vi "Change AO Gain On Fly or Not On Fly.vi"() -> ()   [LabVIEW 2015]
doc: "I. Description:\nThis example demonstrates how to output a continuous periodic waveform using an internal sample clock.\n\nII. Instructions for Running:\n1. Select the Physical Channel to correspond to where your signal is output on the DAQ device.\n2. Enter the Minimum and Maximum Voltage Ranges\n3. Specify the Desired Frequency of the output Waveform\n4. Enter the Waveform Information. See the documentation of the Waveform Buffer Generation SubVI for information on each parameter.\n\nIII. Block Diagram Steps:\n1. Create an Analog Output Voltage channel.\n2. Call the DAQmx Timing (Use Waveform) VI which sets the sample clock rate based on the input waveform parameters, and set the sample mode to Continuous.\n3. Write the waveform to the output buffer.\n4. Call the Start VI.\n5. Loop continuously until the user presses the Stop button. Check for errors every 100 ms using the Is Task Done? VI\n6. Clear the Task\n7. Use the popup dialog box to display an error or warning if any.\n\nIV. I/O Connections Overview:\nMake sure your signal output terminal matches the Physical Channel I/O Control. For further connection information, refer to your hardware reference manual."
uses:
  <vilib>/DAQmx/create/channels.llb/DAQmx Create Channel (AO-Voltage-Basic).vi
  <vilib>/Utility/error.llb/DialogType.ctl
  <vilib>/DAQmx/configure/timing.llb/DAQmx Timing (Sample Clock).vi
  <vilib>/DAQmx/write.llb/DAQmx Write (Analog 2D DBL NChan NSamp).vi
  <resource>/objmgr/daqmx.rc
panel:
  in  "Gain property node":i32
  in  "physical channels 2":tag="PXI1Slot2/ao0" caption="Output Physical Channels"
  in  "AO Idle State":bool=TRUE
  in  "Gain Setting 2":u16(ring) items=["0 dB Gain"=0, "20 dB Gain"=2, "40 dB Gain"=4]
  in  "AO Channel 2":u16(ring)=1536 items=["AO 0"=1536, "AO 1"=1540]
  in  "AO Channel":u16(ring)=1536 items=["AO 0"=1536, "AO 1"=1540]
  in  "Gain Setting":u16(ring) items=["0 dB Gain"=0, "20 dB Gain"=2, "40 dB Gain"=4]
  out "Resulting Frequency":dbl format="%.2f"
  in  "Cycles per Buffer":i32=5
  in  "Waveform Type":T1(ring)
  in  "Desired Frequency":dbl=1000.0 format="%.2f"
  in  "Samples per Buffer":dbl=250.0
  in  "Amplitude":dbl=1750000000.0 format="%0.2p"
  out "Waveform Graph":dbl[](graph) caption="Output Waveform"
  in  "Physical Channels":tag="PXI1Slot2/ao0:1"
  in  "Minimum Value":dbl=-10.0 format="%0.2f"
  in  "Maximum Value":dbl=10.0 format="%0.2f"
  in  "stop":bool
  # "For instructions, select Help>>Show Context Help"
  # "Channel Parameters"
  # "Timing Parameters"
  # "Waveform Information"
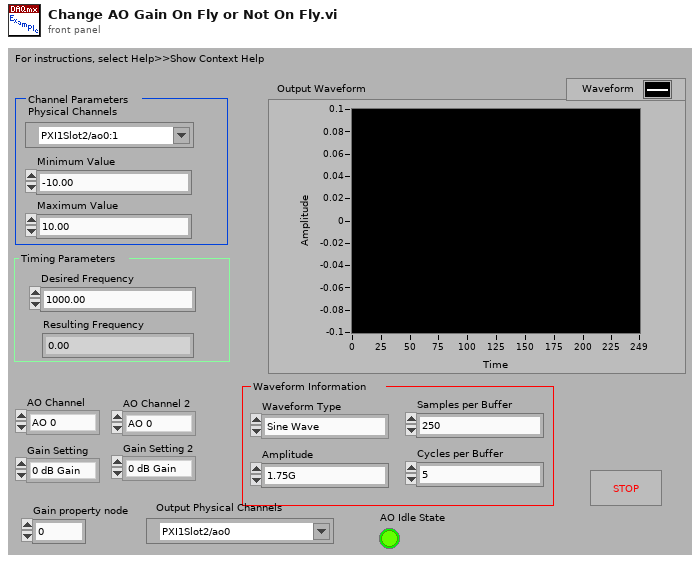
[diagram p1: front panel]
types:
  T1 = enum16{"Sine Wave", "Triangle Wave", "Square Wave", "Sawtooth Wave"}
  T2 = typedef "DialogType.ctl" = u16
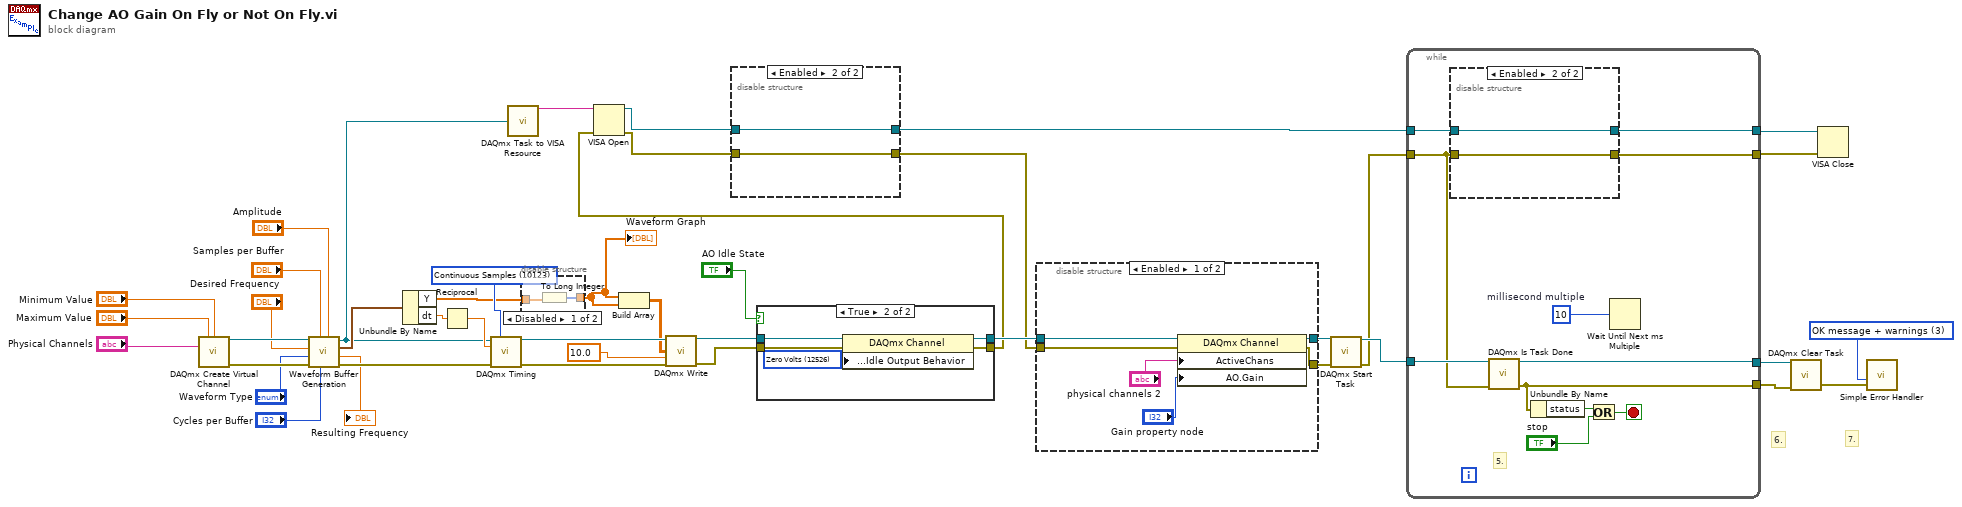
[diagram p0: block diagram]
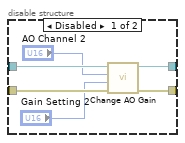
[diagram p5: hidden frame]
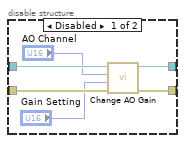
[diagram p6: hidden frame]
diagram:
  w18 = 10123 items=["Finite Samples"=10178, "Continuous Samples"=10123, "Hardware Timed Single Point"=12522] ("sample mode")
  w35 = T2 3 items=["no dialog", "OK message", "continue or stop message", "OK message + warnings", "continue/stop + warnings"] ("type of dialog (OK msg:1)")
  # "7."
  # "6."
  n1 = call-poly <vilib>:"DAQmx Create Virtual Channel.vi"("maximum value"="Maximum Value", "minimum value"="Minimum Value", "physical channels"="Physical Channels") -> ("task out"=w31:refnum<k21>, "error out"=w30:errorcluster)  [unwired: 11 in]
  n2 = call "Waveform Buffer Generation.vi"("Amplitude"="Amplitude", "Cycles per Buffer"="Cycles per Buffer", "Samples per Buffer"="Samples per Buffer", "error in (no error)"=w30, "Waveform Type"="Waveform Type", "Desired Frequency"="Desired Frequency", "task/channels in"=w31) -> ("error out"=w32:errorcluster, "Resulting Frequency"=→"Resulting Frequency":dbl, "Waveform"=w21:waveform(dbl), "task out"=w13:refnum<k21>)  [unwired: 1 out]
  n3 = Unbundle By Name(w21) -> ("Y"=w14:dbl[], "dt"=w20:dbl)
  n4 = Reciprocal(x=w20) -> (1/x=w19:dbl)
  n5 = call-poly <vilib>:"DAQmx Timing.vi"("task/channels in"=w13, "sample mode"=w18, "rate"=w19, "error in"=w32) -> ("task out"=w38:refnum<k21>, "error out"=w37:errorcluster)  [unwired: 10 in]
  n6 = call "DAQmx Task to VISA Resource.vi"("task out"=w13) -> ("VISAName"=w24:string)
  n7 = disable-structure shown="Disabled" {
    disable-tunnel: [w45 w46] -> w15
    disable-tunnel: w14 -> [w44 w46]
    frame Disabled {
      n8 = To Long Integer(number=w44) -> (32bit integer=w45:i32[])
    }
    frame Enabled {
    }
  }
  "Waveform Graph" <- w15
  n9 = Build Array(w15, w15) -> (w17:dbl[][])
  n10 = call-poly <vilib>:"DAQmx Write.vi"("task/channels in"=w38, "data"=w17, "timeout"=10.0 ("Wirite Timeout"), "error in"=w37) -> ("task out"=w11:refnum<k21>, "error out"=w10:errorcluster)  [unwired: 9 in, 1 out]
  n11 = case shown="True" "AO Idle State" {
    tunnel: w11 -> [w48 w53]
    tunnel: w10 -> [w47 w52]
    tunnel: [w48 w51] -> w6
    tunnel: [w47 w50] -> w3
    frame False {
    }
    frame True {
      w49 = 12526 items=["Zero Volts"=12526, "High Impedance"=12527, "Maintain Existing Value"=12528] ("AO.IdleOutputBehavior")
      n12 = property class="DAQmx Channel"(reference=w53, error in=w52, "Analog Output:General Properties:Output Configuration:Idle Output Behavior"=w49) -> (reference out=w51:refnum<k21>, error out=w50:errorcluster)
    }
  }
  n13 = VISA Open(error in (no error)=w3, VISA resource name=w24) -> (VISA resource name=w8:refnum<visa-resource-name>, error out=w7:errorcluster)  [unwired: 3 in]
  n14 = disable-structure shown="Enabled" {
    disable-tunnel: w8 -> [w59 w61]
    disable-tunnel: w7 -> [w58 w60]
    disable-tunnel: [w57 w61] -> w9
    disable-tunnel: [w56 w60] -> w2
    frame Disabled {
      n15 = call "Change AO Gain.vi"("error in"=w58, "Gain Setting"="Gain Setting 2", "AO Channel"="AO Channel 2", "VISA resource name 2"=w59) -> ("error out"=w56:errorcluster, "VISA resource name"=w57:refnum<visa-resource-name>)  [unwired: 4 in]
    }
    frame Enabled {
    }
  }
  n16 = disable-structure shown="Enabled" {
    disable-tunnel: w2 -> [w65 w68]
    disable-tunnel: w6 -> [w64 w69]
    disable-tunnel: [w63 w69] -> w5
    disable-tunnel: [w62 w68] -> w4
    frame Enabled {
      n17 = property class="DAQmx Channel"(reference=w64, error in=w65, "ActiveChans"="physical channels 2", "AO.Gain"="Gain property node") -> (reference out=w63:refnum<k21>, error out=w62:errorcluster)
    }
    frame Disabled {
    }
  }
  n18 = call <vilib>:"DAQmx Start Task.vi"("task/channels in"=w5, "error in"=w4) -> ("task out"=w36:refnum<k21>, "error out"=w1:errorcluster)  [unwired: 12 in]
  n19 = while {
    tunnel: w36 -> [w80]
    tunnel: [w79] -> w34
    tunnel: [w78] -> w33
    tunnel: w9 -> [w73]
    tunnel: w1 -> [w70]
    tunnel: [w72] -> w23
    tunnel: [w71] -> w22
    stop <- w76 stop-if-true
    w77 = u32 10  # millisecond multiple
    # "5."
    n20 = disable-structure shown="Enabled" {
      disable-tunnel: w73 -> [w86 w88]
      disable-tunnel: w70 -> [w85 w87]
      disable-tunnel: [w84 w88] -> w72
      disable-tunnel: [w83 w87] -> w71
      frame Disabled {
        n21 = call "Change AO Gain.vi"("error in"=w85, "Gain Setting"="Gain Setting", "AO Channel"="AO Channel", "VISA resource name 2"=w86) -> ("error out"=w83:errorcluster, "VISA resource name"=w84:refnum<visa-resource-name>)  [unwired: 4 in]
      }
      frame Enabled {
      }
    }
    n22 = call <vilib>:"DAQmx Is Task Done.vi"("task/channels in"=w80, "error in"=w70) -> ("task out"=w79:refnum<k21>, "error out"=w78:errorcluster)  [unwired: 11 in, 1 out]
    n23 = Unbundle By Name(w78) -> ("status"=w75:bool)
    n24 = Or(x=w75, y="stop") -> (x .or. y?=w76:bool)
    n25 = Wait Until Next ms Multiple(millisecond multiple=w77) -> ()  [unwired: 1 out]
  }
  n26 = call <vilib>:"DAQmx Clear Task.vi"("task in"=w34, "error in"=w33) -> ("error out"=w43:errorcluster)  [unwired: 13 in]
  n27 = VISA Close(VISA resource name=w23, error in (no error)=w22) -> ()  [unwired: 1 out]
  n28 = call <vilib>:"Simple Error Handler.vi"("type of dialog (OK msg:1)"=w35, "error in (no error)"=w43) -> ()  [unwired: 3 in, 5 out]
